vi "CalcTempHumidity.vi"(11 "Data":string) -> (2 "Temperature (°C)":dbl, 3 "RHumidity%":dbl)   [LabVIEW 2024]
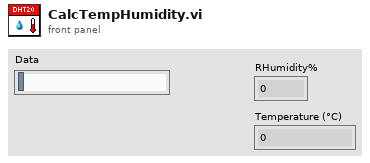
[diagram p1: front panel]
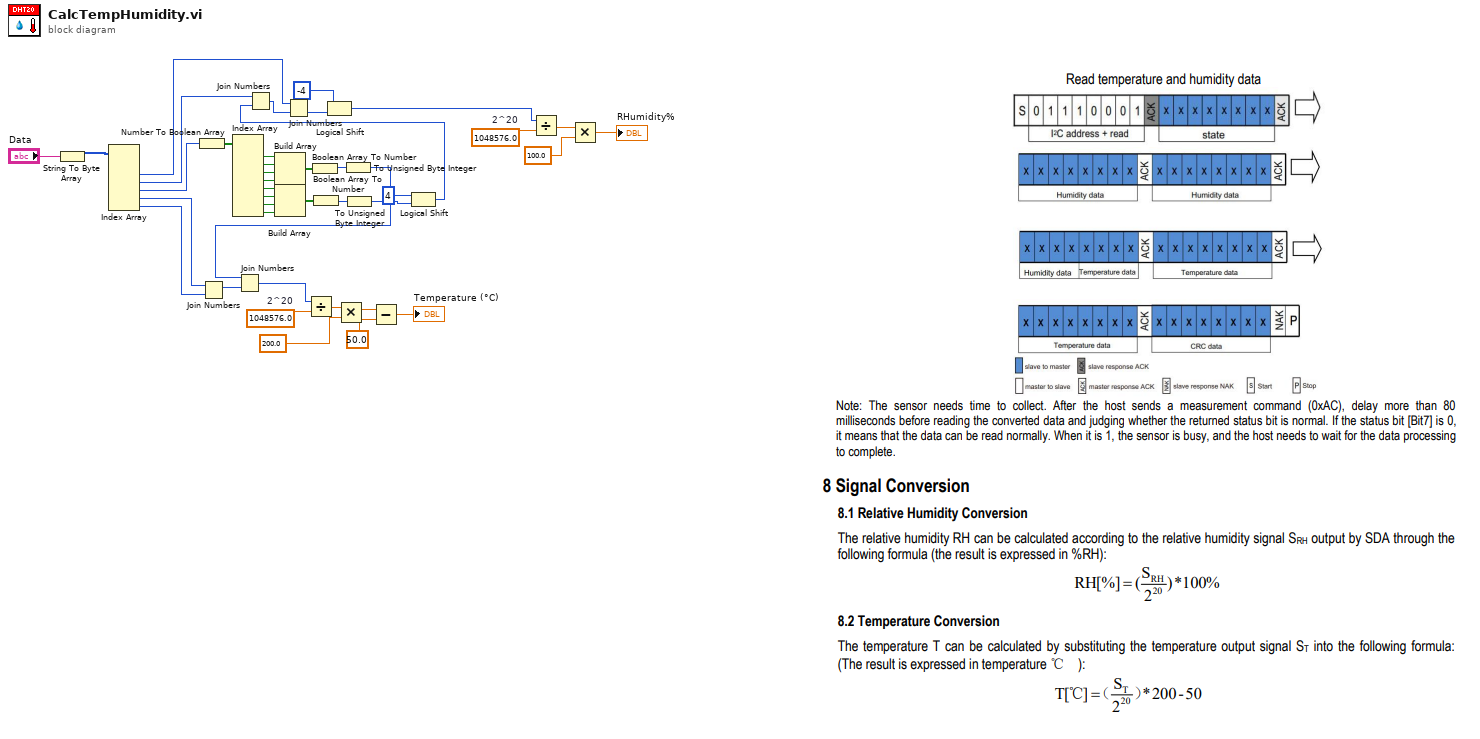
[diagram p0: block diagram]
diagram:
  w36 = 1048576.0  # 2^20
  w37 = 1048576.0  # 2^20
  n1 = String To Byte Array(string="Data") -> (unsigned byte array=w39:u8[])
  n2 = Index Array(array=w39) -> (element #2=w9:u8, element #3=w8:u8, element #4=w25:u8, element #5=w27:u8, element #6=w26:u8)  [unwired: 6 in, 1 out]
  n3 = Number To Boolean Array(number=w25) -> (Boolean array=w24:bool[])
  n4 = Join Numbers(hi=w27, lo=w26) -> ((hi.lo)=w38:u16)
  n5 = Index Array(array=w24) -> (element #1=w23:bool, element #2=w22:bool, element #3=w21:bool, element #4=w20:bool, element #5=w19:bool, element #6=w18:bool, element #7=w17:bool, element #8=w16:bool)  [unwired: 8 in]
  n6 = Build Array(w23, w22, w21, w20) -> (w15:bool[])
  n7 = Build Array(w19, w18, w17, w16) -> (w14:bool[])
  n8 = Boolean Array To Number(Boolean array=w15) -> (number=w13:u32)
  n9 = Boolean Array To Number(Boolean array=w14) -> (number=w12:u32)
  n10 = To Unsigned Byte Integer(number=w13) -> (unsigned 8bit integer=w11:u8)
  n11 = Join Numbers(hi=w11, lo=w38) -> ((hi.lo)=w1:u32)
  n12 = Divide(x=w1, y=w37) -> (x/y=w35:dbl)
  n13 = Multiply(x=w35, y=200.0) -> (x*y=w33:dbl)
  n14 = To Unsigned Byte Integer(number=w12) -> (unsigned 8bit integer=w7:u8)
  n15 = Subtract(x=w33, y=50.0) -> (x-y=→"Temperature (°C)":dbl)
  n16 = Logical Shift(y=i16 4, x=w7) -> (x << y=w6:u8)
  n17 = Join Numbers(hi=w8, lo=w6) -> ((hi.lo)=w10:u16)
  n18 = Join Numbers(hi=w9, lo=w10) -> ((hi.lo)=w4:u32)
  n19 = Logical Shift(y=i16 -4, x=w4) -> (x << y=w2:u32)
  n20 = Divide(x=w2, y=w36) -> (x/y=w30:dbl)
  n21 = Multiply(x=w30, y=100.0) -> (x*y=→"RHumidity%":dbl)
